vi "PH_BeamlineInformation.get Head Information by PU.vi"(1 "Heads":T2[](array[typedef]), 4 "Power Unit":T1) -> (14 "In Use?":bool, 15 "In Use linked?":bool, 16 "Applied Voltage":dbl, 17 "Voltage linked?":bool, 18 "In Use GUI Ref":refnum<vi>, 19 "Voltage GUI Ref":refnum<vi>)   [LabVIEW 2014, in "PH_BeamlineInformation.lvlib"]
uses:
  PH_BeamlineInformation.lvlib
  PH_BeamlineInformation.Head.ctl
  PH_PP_Common/PH_PP_Common.PUs.ctl
  PH_PP_Common/PH_PP_Common.lvlib
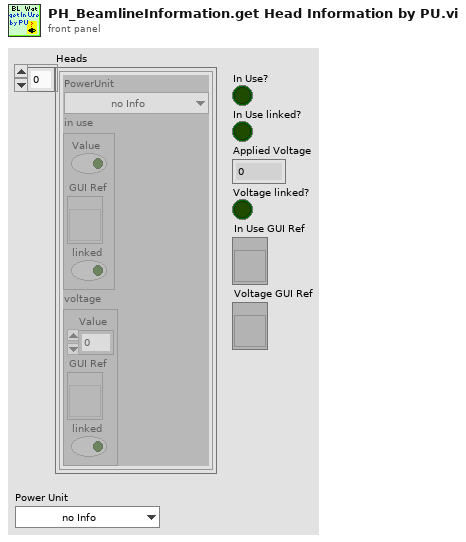
[diagram p1: front panel]
types:
  T1 = typedef "PH_PP_Common.lvlib/PH_PP_Common.PUs.ctl" = enum16{"no Info", "PA-19mm-1", "PA-19mm-2", "PA-45mm-PILC", "PA-45mm-MAIN", "MA-PU-1", "MA-PU-2", "MA-PU-3", "MA-PU-4", "MA-PU-5", "MA-PU-6", "MA-FR", "MA-PILC", "PA-45mm-DP"}
  T2 = typedef "PH_BeamlineInformation.lvlib/PH_BeamlineInformation.Head.ctl" = cluster{"PowerUnit":T1, "in use":cluster{"Value":bool, "GUI Ref":refnum<vi>, "linked":bool}, "voltage":cluster{"Value":dbl, "GUI Ref":refnum<vi>, "linked":bool}}
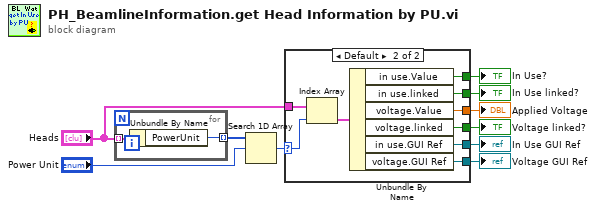
[diagram p0: block diagram]
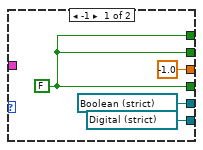
[diagram p2: hidden frame]
diagram:
  n1 = for {
    tunnel: "Heads" -> [w12] mode=indexing
    tunnel: [w11] -> w5 mode=indexing
    n2 = Unbundle By Name(w12) -> ("PowerUnit"=w11:T1)
  }
  n3 = Search 1D Array(1D array=w5, element="Power Unit") -> (index of element=w7:i32)  [unwired: 1 in]
  n4 = case shown="Default" w7 {
    selector: w7 -> [_ w24]
    tunnel: "Heads" -> [_ w25]
    tunnel: [w15 w22] -> w9
    tunnel: [w15 w21] -> w10
    tunnel: [-1.0 ("Value") w20] -> w4
    tunnel: [w15 w19] -> w3
    tunnel: [refnum<vi> refnum ("GUI Ref") w18] -> w2
    tunnel: [refnum<vi> refnum ("GUI Ref") w17] -> w1
    frame -1 {
      w15 = FALSE ("Value")
    }
    frame Default {
      n5 = Index Array(array=w25, index=w24) -> (element=w23:T2)
      n6 = Unbundle By Name(w23) -> ("in use.Value"=w22:bool, "in use.linked"=w21:bool, "voltage.Value"=w20:dbl, "voltage.linked"=w19:bool, "in use.GUI Ref"=w18:refnum<vi>, "voltage.GUI Ref"=w17:refnum<vi>)
    }
  }
  "In Use?" <- w9
  "In Use linked?" <- w10
  "Applied Voltage" <- w4
  "Voltage linked?" <- w3
  "In Use GUI Ref" <- w2
  "Voltage GUI Ref" <- w1
